vi "_Hightlight CSM Scripts(StringControl).vi"(11 "String Ctrl":refnum<vi>) -> ()   [LabVIEW 2017]
uses:
  Communicable State Machine.lvlib
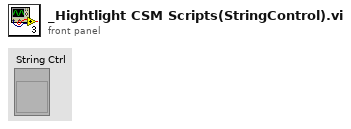
[diagram p1: front panel]
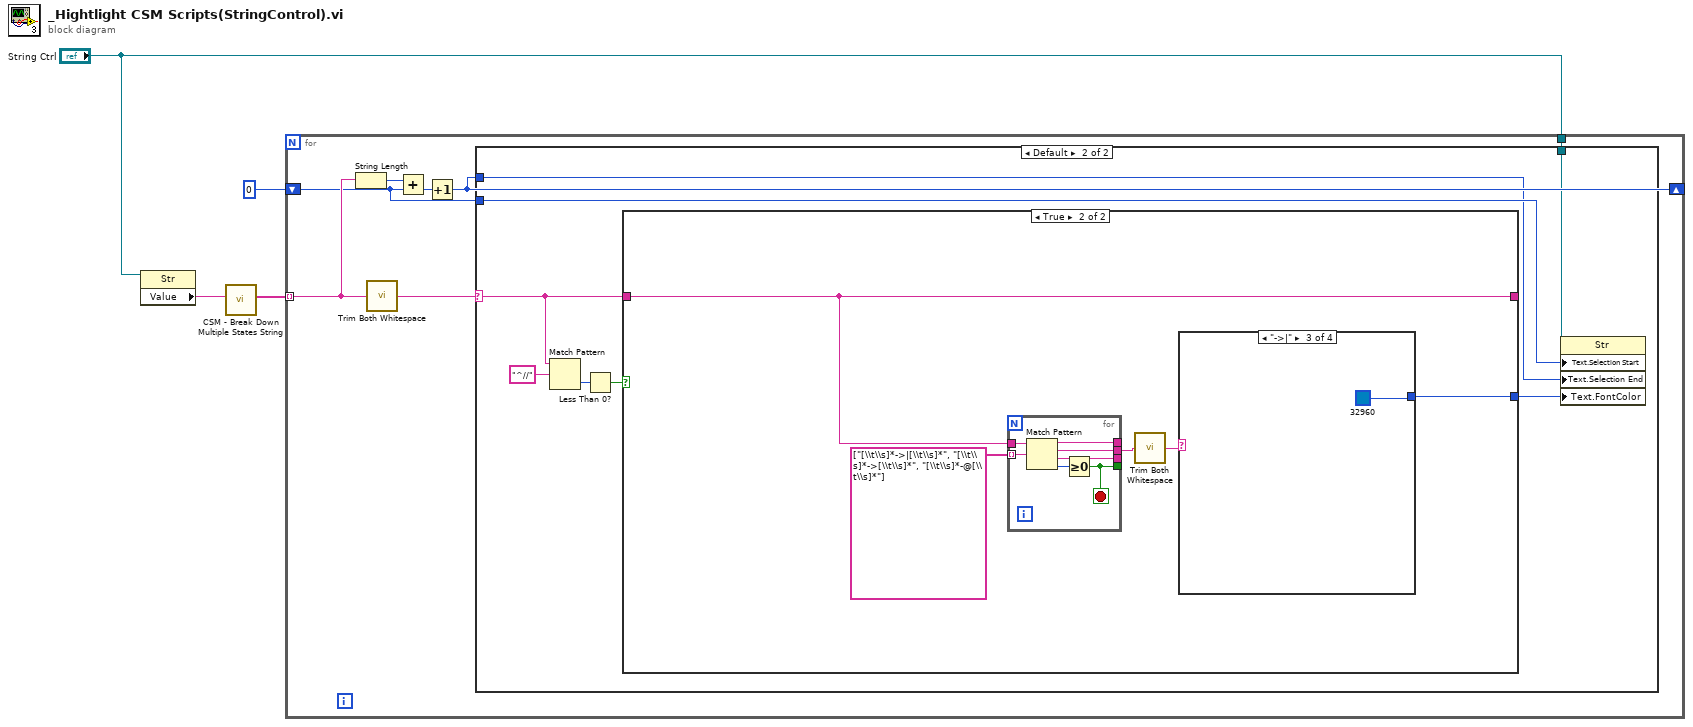
[diagram p0: block diagram]
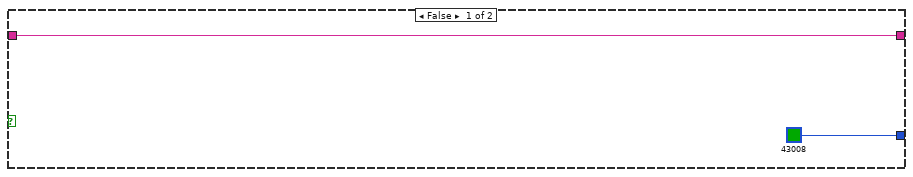
[diagram p3: hidden frame]
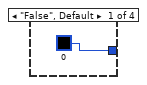
[diagram p4: hidden frame]
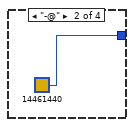
[diagram p5: hidden frame]
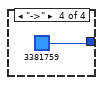
[diagram p6: hidden frame]
diagram:
  n1 = property class="Str"(reference="String Ctrl") -> ("Value"=w2:string)  [unwired: 1 in, 2 out]
  n2 = call "CSM - Break Down Multiple States String.vi"("States"=w2) -> ("Multiple States"=w4:string[])  [unwired: 10 in]
  n3 = for {
    tunnel: w4 -> [w9] mode=indexing
    shift-right: [w5] -> _
    shift-left: u32 0 ("Text.Selection:Start") -> [w7]
    tunnel: "String Ctrl" -> [w8]
    n4 = String Length(string=w9) -> (length=w10:i32)
    n5 = call "Trim Both Whitespace.vi"("string"=w9) -> ("trimmed string"=w11:string)  [unwired: 1 in]
    n6 = Add(x=w10, y=w7) -> (x+y=w6:u32)
    n7 = Increment(x=w6) -> (x+1=w5:u32)
    n8 = case shown="Default" w11 {
      selector: w11 -> [_ w17]
      tunnel: w8 -> [_ w15]
      tunnel: w7 -> [_ w14]
      tunnel: w5 -> [_ w13]
      frame "" {
      }
      frame Default {
        n9 = Match Pattern(string=w17, regular expression="^//") -> (offset past match=w19:i32)  [unwired: 1 in, 3 out]
        n10 = Less Than 0?(x=w19) -> (x < 0?=w16:bool)
        n11 = case shown="True" w16 {
          tunnel: [w21 w24] -> _
          tunnel: w17 -> [w21 w24]
          tunnel: [u32 43008 w23] -> w12
          frame False {
          }
          frame True {
            n12 = for {
              tunnel: w24 -> [w37]
              tunnel: string[] ["[\\t\\s]*->|[\\t\\s]*", "[\\t\\s]*->[\\t\\s]*", "[\\t\\s]*-@[\\t\\s]*"] -> [w36] mode=indexing
              tunnel: [w34] -> _
              tunnel: [w33] -> _
              tunnel: [w32] -> w25
              tunnel: [w31] -> _
              stop <- w34 stop-if-true
              n13 = Match Pattern(string=w37, regular expression=w36) -> (before substring=w33:string, match substring=w32:string, after substring=w31:string, offset past match=w35:i32)  [unwired: 1 in]
              n14 = Greater Or Equal To 0?(x=w35) -> (x >= 0?=w34:bool)
            }
            n15 = call "Trim Both Whitespace.vi"("string"=w25) -> ("trimmed string"=w22:string)  [unwired: 1 in]
            n16 = case shown="\"->|\"" w22 {
              tunnel: [u32 0 u32 14461440 u32 32960 u32 3381759] -> w23
              frame "False", Default {
              }
              frame "-@" {
              }
              frame "->|" {
              }
              frame "->" {
              }
            }
          }
        }
        n17 = property class="Str"(reference=w15, "Text.Selection Start"=w14, "Text.Selection End"=w13, "Text.FontColor"=w12) -> ()  [unwired: 1 in, 2 out]
      }
    }
  }
